vi "COMM Write TX message.vi"(10 "data":variant, 11 "parameters":string) -> (0 "error out":T1)   [LabVIEW 2019, in "Communication Interface.lvlib"]
uses:
  Communication Interface.lvlib
  SubVIs/Shared/CMD Write tx.ctl
  SubVIs/mmWave HW Control/HW custom error.ctl
  be307184-fad8-4add-a6ed-4e685d635292.vi
  be307184-fad8-4add-a6ed-4e685d635292.vi/34c215fd-40ee-4e18-b44d-a745019a197e.vi
  be307184-fad8-4add-a6ed-4e685d635292.vi/a1c05146-a897-4c5e-af07-17c754f605b2.vi
  <vilib>/Utility/High Resolution Relative Seconds.vi
  <vilib>/Utility/error.llb/Clear Errors.vi
  SubVIs/IQBurst_memo_class/IQBurst_memo.lvclass
  C:/Barkhausen mmWave radar/Development/LV/Barkhausen mmWave hardware control/Host/SubVIs/mmWave data_class/mmWave data.lvclass
  <vilib>/addons/_JKI.lib/Serialization/JSON/Library/Unflatten From JSON String.vi
  SubVIs/Shared/Shared.lvlib
  SubVIs/mmWave HW Control/mmWave HW Control.lvlib
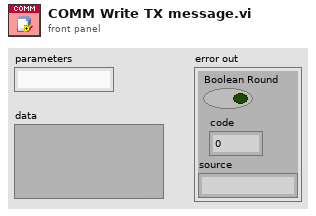
[diagram p1: front panel]
types:
  T1 = cluster{"Boolean Round":bool, "code":i32, "source":string}
  T2 = typedef "mmWave HW Control.lvlib/HW custom error.ctl" = u16
  T3 = typedef "Shared.lvlib/CMD Write tx.ctl" = cluster{"burst name":string}
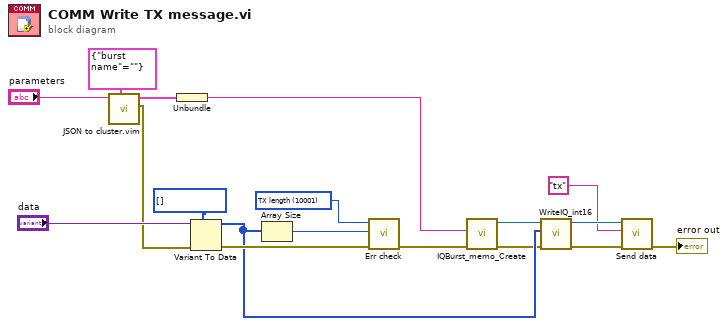
[diagram p0: block diagram]
diagram:
  w17 = T2 10001 items=["TX list"=10000, "TX length"=10001, "RX length"=10002] ("HW custom err")
  n1 = call "JSON to cluster.vim"("data"=T3 {"burst name"=""} ("write tx command"), "JSON in"="parameters") -> ("error out"=w1:errorcluster, "data"=w9:T3)  [unwired: 7 in, 1 out]
  n2 = Unbundle(w9) -> ("burst name"=w13:string)
  n3 = Variant To Data(error in=w1, type=i16[] [] ("TX.IQ signal"), Variant="data") -> (data=w15:i16[], error out=w18:errorcluster)
  n4 = Array Size(array=w15) -> (size(s)=w16:i32)
  n5 = call "Err check.vi"("error in"=w18, "Variant Control"=w16, "HW custom err"=w17) -> ("error out"=w4:errorcluster)  [unwired: 8 in]
  n6 = call "IQBurst_memo_Create.vi"("error in (no error)"=w4, "burst name"=w13) -> ("error out"=w3:errorcluster, "reference out"=w12:refnum<class "IQBurst_memo.lvclass">)  [unwired: 8 in]
  n7 = call-dynamic "WriteIQ_int16.vi"("error in (no error)"=w3, "data"=w15, "reference in"=w12) -> ("error out"=w2:errorcluster, "reference out"=w14:refnum<class "IQBurst_memo.lvclass">)  [unwired: 7 in]
  n8 = call "Send data.vi"("error in (no error)"=w2, "group"="tx", "Data"=w14) -> ("error out"=→"error out":T1)  [unwired: 8 in]
